vi "timer.vi"(8 "error in (no error)":errorcluster, 10 "timerstatus":T1, 11 "limit":dbl) -> (0 "error out":errorcluster, 2 "elapsed":dbl, 3 "out of limit":bool)   [LabVIEW 2015]
uses:
  timerstatus.ctl
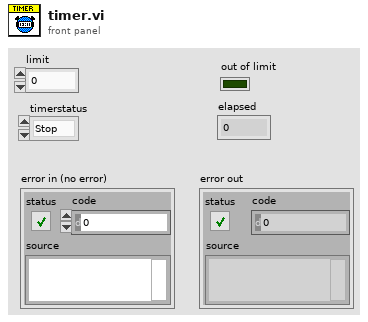
[diagram p1: front panel]
types:
  T1 = typedef "timerstatus.ctl" = enum16{"Stop", "Start"}
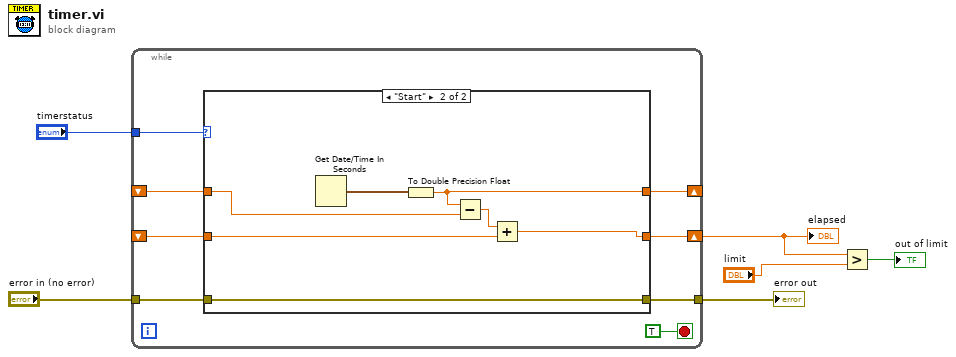
[diagram p0: block diagram]
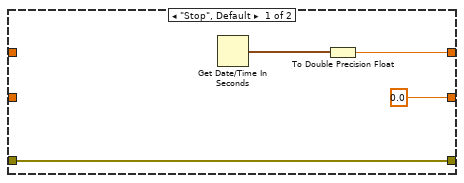
[diagram p2: hidden frame]
diagram:
  n1 = while {
    tunnel: "timerstatus" -> [w14]
    shift-right: [w13] -> _
    shift-left: _ -> [w8]
    shift-right: [w12] -> w2
    shift-left: _ -> [w7]
    tunnel: "error in (no error)" -> [w11]
    tunnel: [w10] -> w4
    stop <- TRUE stop-if-true
    n2 = case shown="\"Start\"" w14 {
      tunnel: [w17 w22] -> w13
      tunnel: [0.0 w19] -> w12
      tunnel: w11 -> [w15 w25]
      tunnel: [w15 w25] -> w10
      tunnel: w8 -> [_ w23]
      tunnel: w7 -> [_ w20]
      frame "Stop", Default {
        n3 = Get Date/Time In Seconds() -> (seconds since 1Jan1904=w18:timestamp)
        n4 = To Double Precision Float(number=w18) -> (double precision float=w17:dbl)
      }
      frame "Start" {
        n5 = Get Date/Time In Seconds() -> (seconds since 1Jan1904=w24:timestamp)
        n6 = To Double Precision Float(number=w24) -> (double precision float=w22:dbl)
        n7 = Subtract(x=w22, y=w23) -> (x-y=w21:dbl)
        n8 = Add(x=w21, y=w20) -> (x+y=w19:dbl)
      }
    }
  }
  "error out" <- w4
  "elapsed" <- w2
  n9 = Greater?(x=w2, y="limit") -> (0:→"out of limit":bool)
